vi "Untitled 2.vi"() -> ()   [LabVIEW 2020]
panel:
  out "Tank":u64(slide) scale=0.0..50.0
  in  "Boþalt":dbl(knob) scale=0.0..10.0
  in  "Doldur":dbl(knob) scale=0.0..10.0
  # "Ahmed Göktuð Aydýn - 200208054"
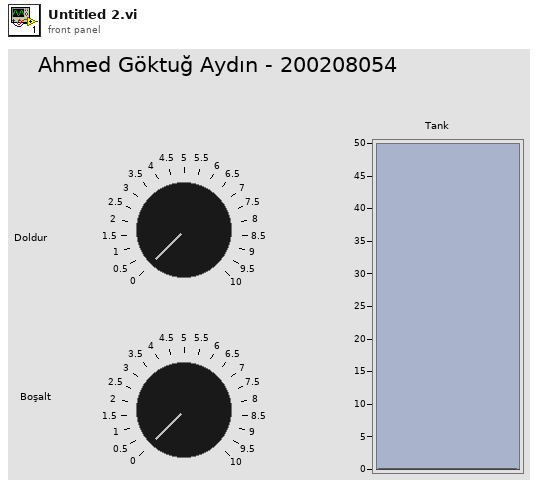
[diagram p1: front panel]
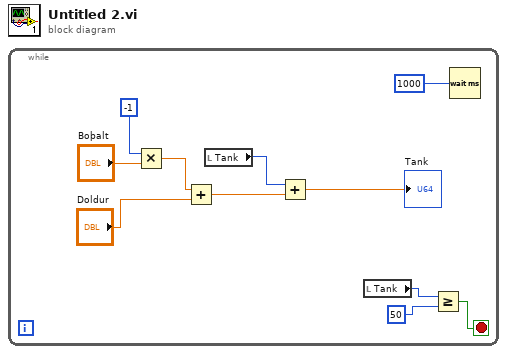
[diagram p0: block diagram]
diagram:
  n1 = while {
    stop <- w4 stop-if-true
    n2 = Multiply(x=-1, y="Boþalt") -> (x*y=w10:dbl)
    n3 = Add(x=w10, y="Doldur") -> (x+y=w11:dbl)
    n4 = local read "Tank"() -> (w1:u64)
    n5 = Add(x=w1, y=w11) -> (x+y=→"Tank":dbl)
    n6 = local read "Tank"() -> (w3:u64)
    n7 = Greater Or Equal?(x=w3, y=50) -> (x >= y?=w4:bool)
    n8 = Wait (ms)(milliseconds to wait=1000) -> ()  [unwired: 1 out]
  }
